vi "ReadIVIsamplescope.vi"(5 "channel name (\"CHANNEL1\")":string="CHANNEL1", 6 "instrument handle":refnum<k15>) -> (0 "error out":errorcluster {"code" format="%.0x"}, 1 "waveform array":dbl[](array[numeric]) format="%.3f", 2 "actual points":i32, 3 "instrument handle out":refnum<k15>, 4 "x increment":dbl caption="x increment (seconds)" format="%^.2e")   [LabVIEW 2011]
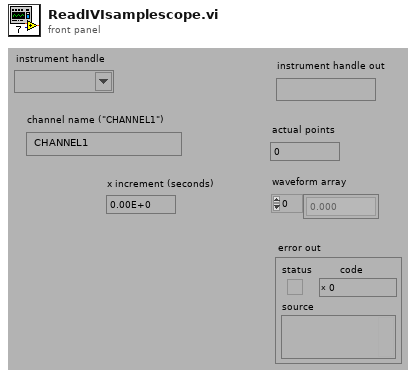
[diagram p1: front panel]
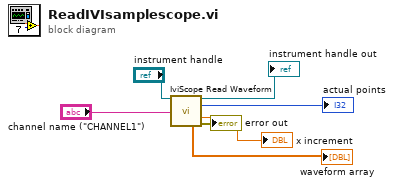
[diagram p0: block diagram]
diagram:
  n1 = call <vilib>:"IviScope Read Waveform.vi"("instrument handle"="instrument handle", "channel name (\"CHANNEL1\")"="channel name (\"CHANNEL1\")") -> ("instrument handle out"=→"instrument handle out":refnum<k15>, "actual points"=→"actual points":i32, "x increment"=→"x increment":dbl, "waveform array"=→"waveform array":dbl[], "error out"=→"error out":errorcluster)  [unwired: 3 in, 6 out]
